vi "Set Valve Position.vi"(8 "error in (no error)":errorcluster, 10 "Valve Pos":u16, 11 "Autosampler in":refnum<class "Autosampler.lvclass">) -> (0 "error out":errorcluster, 3 "Autosampler out":refnum<class "Autosampler.lvclass">)   [LabVIEW 2023, in "Autosampler.lvlib" / "Autosampler.lvclass"]
uses:
  Autosampler.lvclass
  Autosampler.lvclass/Autosampler.ctl
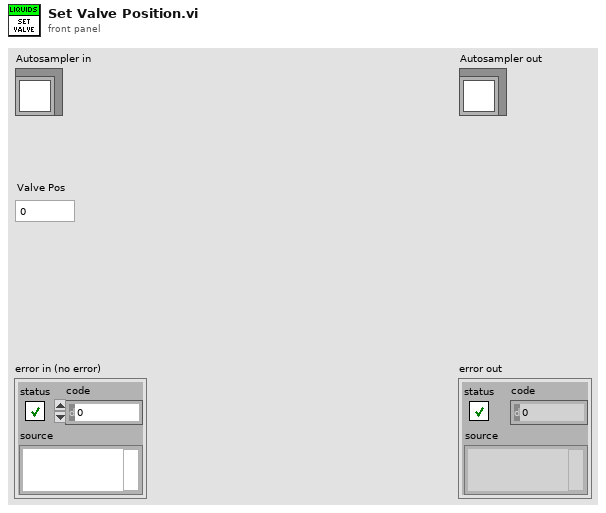
[diagram p1: front panel]
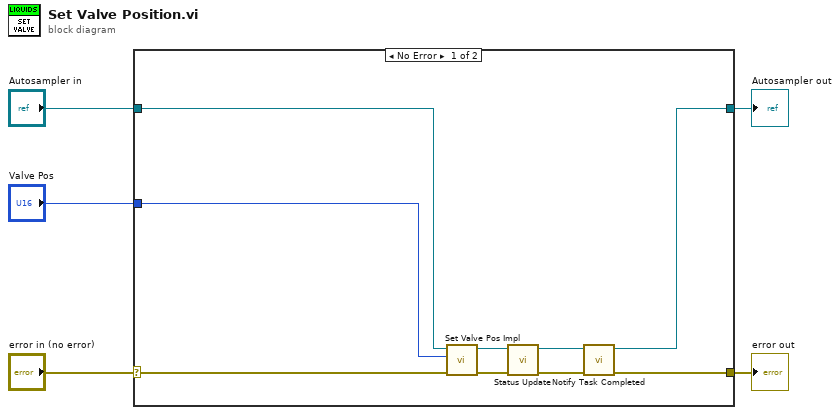
[diagram p0: block diagram]
diagram:
  n1 = case shown="No Error" "error in (no error)" {
    selector: "error in (no error)" -> [w14 w16]
    tunnel: [w6 w16] -> w4
    tunnel: [w7 w15] -> w2
    tunnel: "Autosampler in" -> [w13 w15]
    tunnel: "Valve Pos" -> [w12 _]
    frame No Error {
      n2 = call-dynamic "Set Valve Pos Impl.vi"("error in (no error)"=w14, "Valve Pos"=w12, "Autosampler in"=w13) -> ("error out"=w11:errorcluster, "Autosampler out"=w10:refnum<class "Autosampler.lvclass">)  [unwired: 7 in]
      n3 = call "Status Update.vi"("error in (no error)"=w11, "Autosampler in"=w10) -> ("error out"=w9:errorcluster, "Autosampler out"=w8:refnum<class "Autosampler.lvclass">)  [unwired: 8 in]
      n4 = call-dynamic "Notify Task Completed.vi"("error in (no error)"=w9, "Device in"=w8) -> ("error out"=w6:errorcluster, "Device out"=w7:refnum<class "Autosampler.lvclass">)  [unwired: 8 in]
    }
    frame Error {
    }
  }
  "error out" <- w4
  "Autosampler out" <- w2
